vi "MetaData Channel.vi"(8 "error in (no error)":errorcluster, 11 "Node Ptr":T5 format="%.0x") -> (0 "error out":errorcluster)   [LabVIEW 2019, in "Instrument Addon System Explorer.lvlib"]
uses:
  Instrument Addon System Explorer.lvlib
  <vilib>/NI VeriStand/Custom Device API/Custom Device API.lvlib
  Addon Shared/Instrument Addon Shared.lvlib
  Addon Shared/Types/FG Control.ctl
  <vilib>/NI VeriStand/Custom Device API/Custom Device Channel Type.ctl
  <vilib>/NI VeriStand/Custom Device API/Custom Device Channel.ctl
  Addon Shared/Constants.vi
  <vilib>/NI VeriStand/Custom Device API/Custom Device Item Ref.ctl
  Addon Shared/Types/Protocol Data Type.ctl
  Addon Shared/Types/Metadata Channel Type.ctl
  Addon Shared/Types/Type Cast Type.ctl
  Addon Shared/Types/Endian.ctl
panel:
  in  "Delimiter":string=","
  in  "Reset":bool
  in  "Create":bool
  in  "Elements":u32
  in  "Units":string
  in  "Default Value":dbl
  out "Channel Type (Tab)":enum32{"List", "Format", "Type Cast"}(tab)
  in  "Remove":bool
  in  "Add":bool
  in  "Enumerated List":i32(listbox)
  in  "Test Value":dbl
  in  "Format String":string="%.3g"
  out "Validiated String":string
  in  "Endian":T1=enum."Little"
  in  "Type":T2
  in  "Channel Type":T3
  out "Data Type":T4
  in  "Header 2":cluster{"Section Name":string}={"Section Name"="MetaData Settings"}
  in  "SHDocVw.IWebBrowser":refnum<k7>(container)
  in  "Header":cluster{"Section Name":string}={"Section Name"="Custom Device Item Settings"}
  in  "Description":string
  in  "Name":string
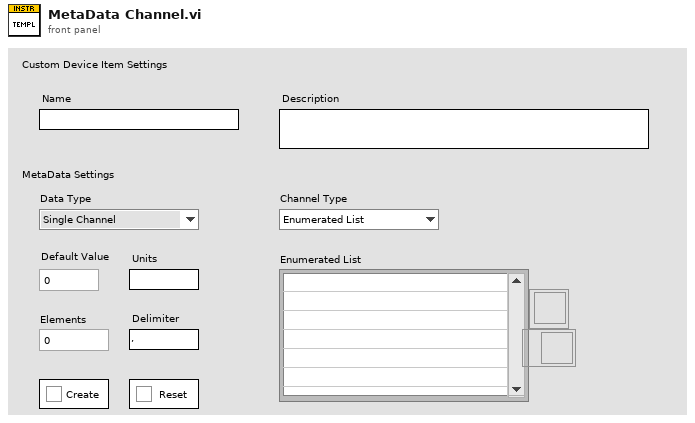
[diagram p1: front panel]
types:
  T1 = typedef "Instrument Addon Shared.lvlib/Endian.ctl" = enum16{"Native", "Little", "Big"}
  T2 = typedef "Instrument Addon Shared.lvlib/Type Cast Type.ctl" = enum16{"DBL", "SGL", "U64", "U32", "U16", "U8", "I64", "I32", "I16", "I8"}
  T3 = typedef "Instrument Addon Shared.lvlib/Metadata Channel Type.ctl" = enum16{"Enumerated List", "Format", "Type Cast"}
  T4 = typedef "Instrument Addon Shared.lvlib/Protocol Data Type.ctl" = enum16{"Single Channel", "Array"}
  T5 = typedef "Custom Device API.lvlib/Custom Device Item Ref.ctl" = u64
  T6 = typedef "Instrument Addon Shared.lvlib/FG Control.ctl" = enum16{"Get", "Set"}
  T7 = typedef "Custom Device API.lvlib/Custom Device Item Info.ctl" = cluster{"Name":string, "Is Channel":bool, "GUID":string, "Is Waveform":bool}
  T8 = typedef "Instrument Addon Shared.lvlib/MetaData Parameters.ctl" = cluster{"Data Type":T4, "Channel Type":T3, "List":string[], "Format String":string, "Type":T2, "Delimiter":string, "Endian":T1}
  T9 = typedef "Custom Device API.lvlib/Custom Device Channel.ctl" = cluster{"Type":T10, "Units":string, "Default Value":dbl, "Faultable":bool, "Scalable":bool}
  T10 = typedef "Custom Device API.lvlib/Custom Device Channel Type.ctl" = enum16{"Input", "Output"}
  T11 = typedef "Custom Device API.lvlib/Custom Device Commands.ctl" = enum16{"Default", "Item renamed", "Shutdown", "Dynamic button pressed"}
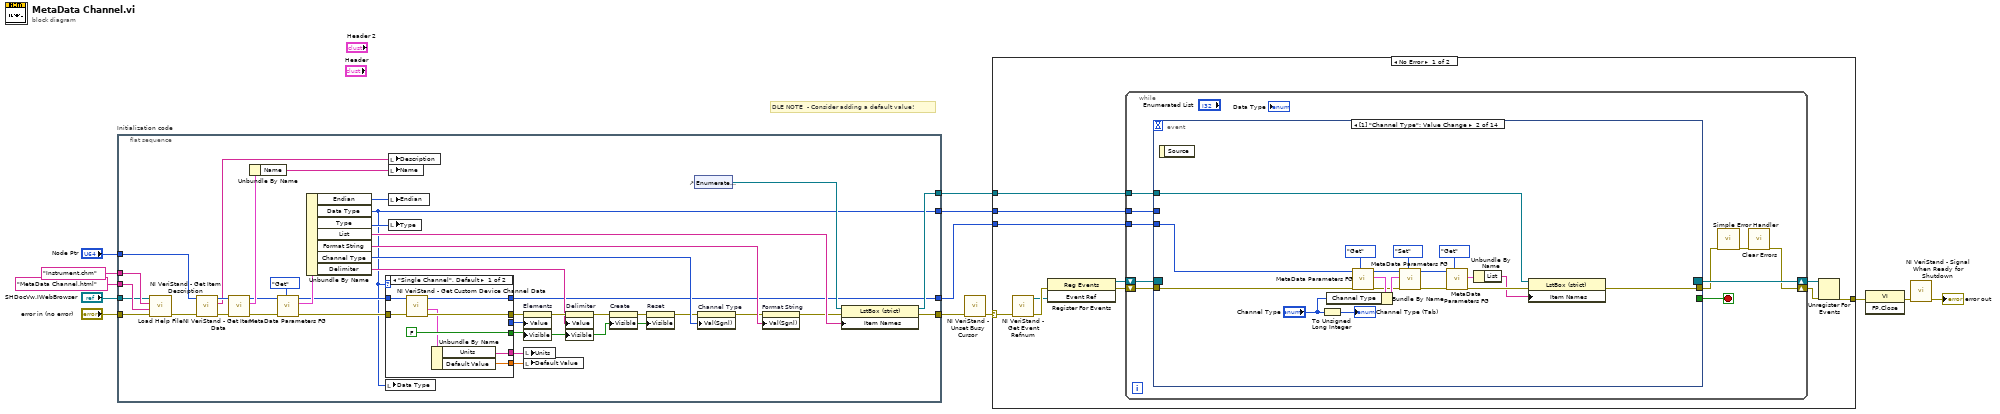
[diagram p0: block diagram]
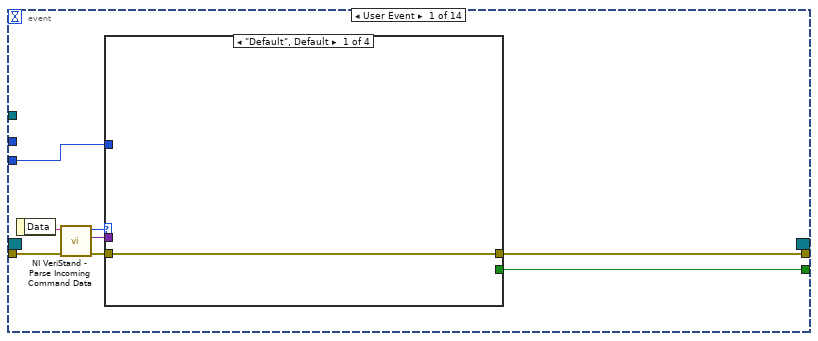
[diagram p2: hidden frame]
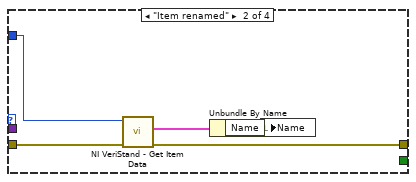
[diagram p3: hidden frame]
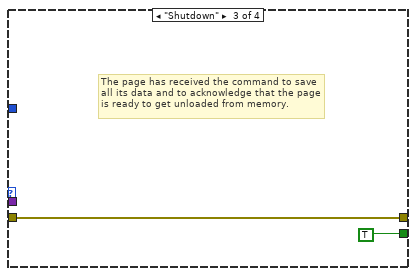
[diagram p4: hidden frame]
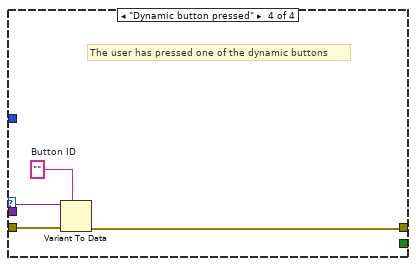
[diagram p5: hidden frame]
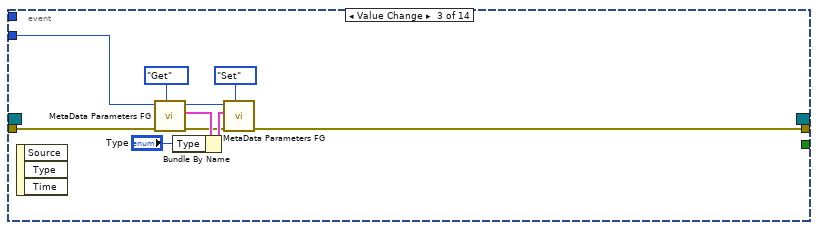
[diagram p6: hidden frame]
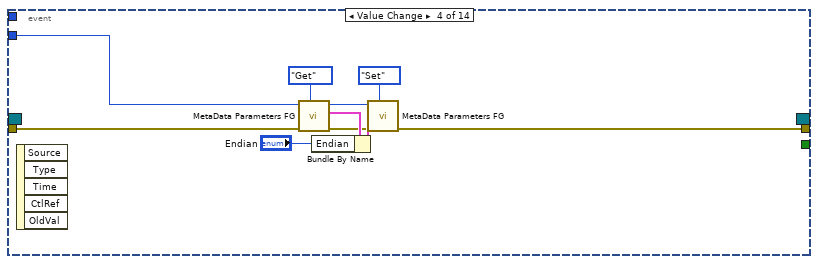
[diagram p7: hidden frame]
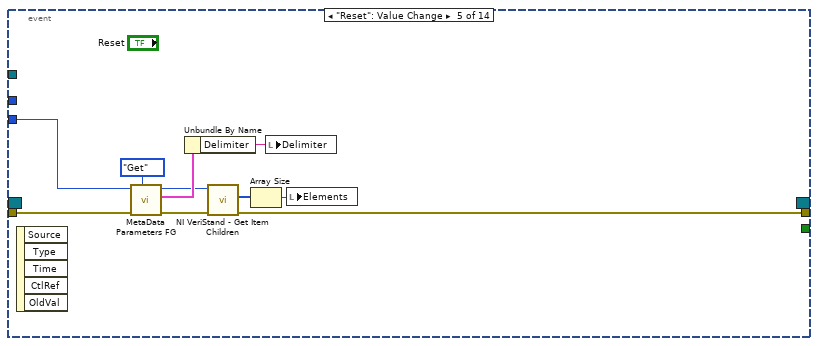
[diagram p8: hidden frame]
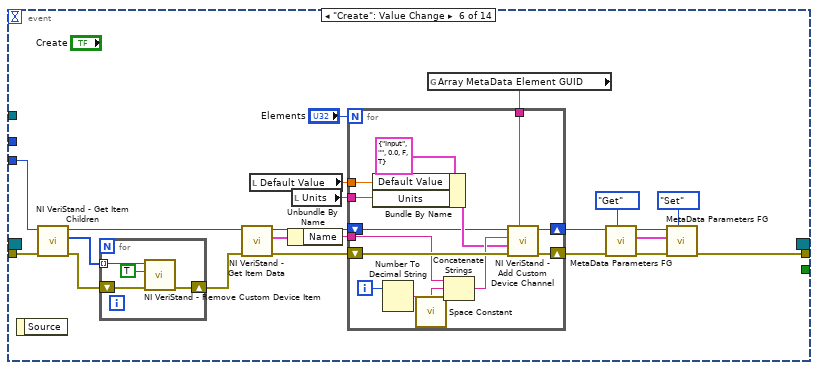
[diagram p9: hidden frame]
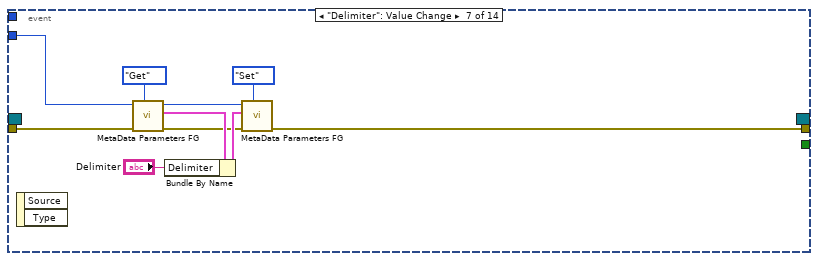
[diagram p10: hidden frame]
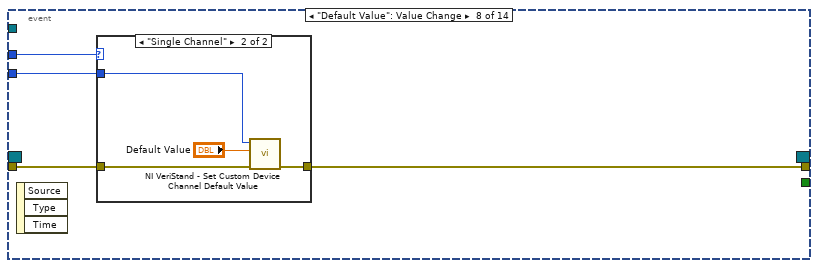
[diagram p11: hidden frame]
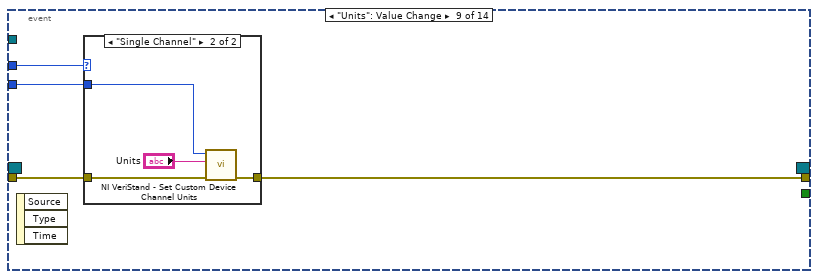
[diagram p13: hidden frame]
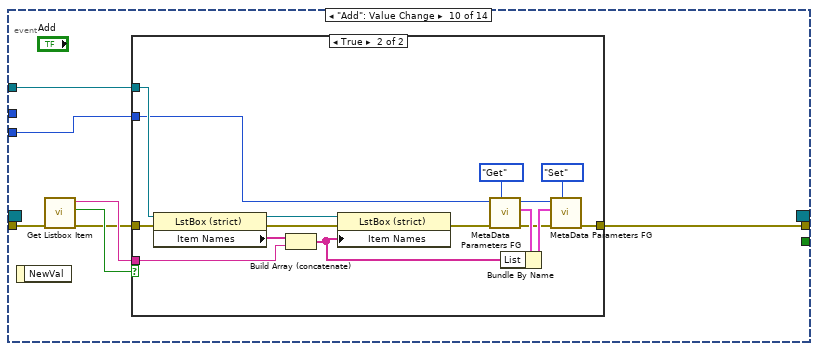
[diagram p15: hidden frame]
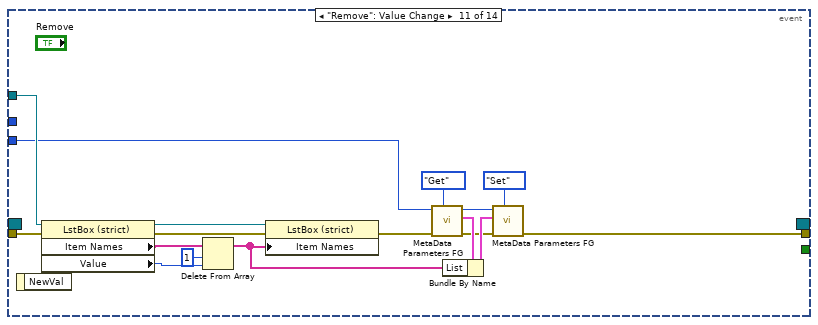
[diagram p17: hidden frame]
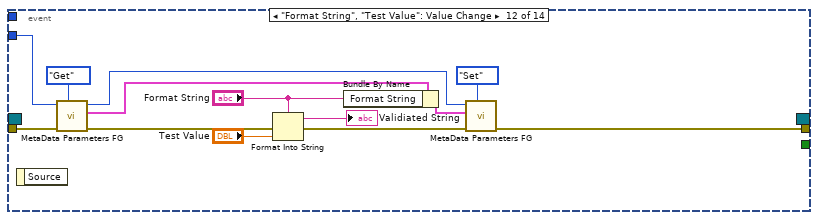
[diagram p18: hidden frame]
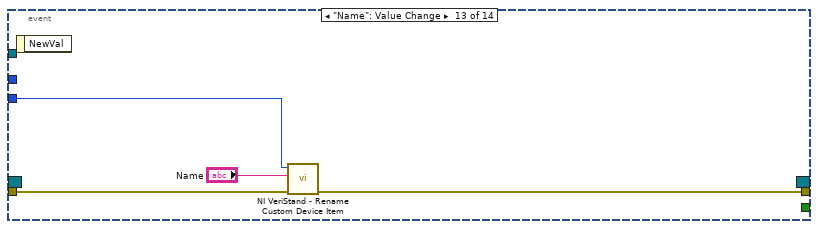
[diagram p19: hidden frame]
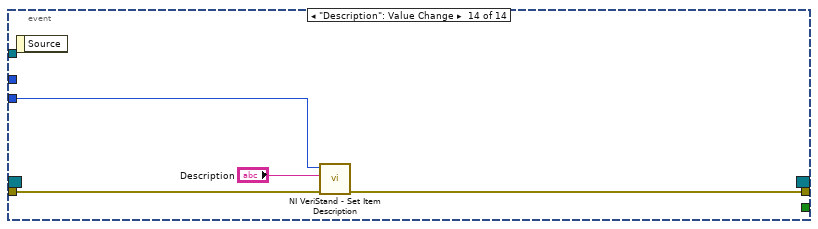
[diagram p20: hidden frame]
diagram:
  # "DLE NOTE  - Consider adding a default value!"
  n1 = flat-sequence "Initialization code" {
    tunnel: "error in (no error)" -> [w47]
    tunnel: "Node Ptr" -> [w32]
    tunnel: [w36] -> w9
    tunnel: [w20] -> w2
    tunnel: "Instrument.chm" ("Main CHM File") -> [w46]
    tunnel: "MetaData Channel.html" ("HTML File") -> [w45]
    tunnel: "SHDocVw.IWebBrowser" -> [w44]
    tunnel: [w34] -> w3
    tunnel: [w17] -> w1
    frame #0 {
      n2 = call "Load Help File.vi"("error in (no error)"=w47, "HTML File"=w45, "Main CHM File"=w46, "SHDocVw.IWebBrowser2"=w44) -> ("error out"=w33:errorcluster)  [unwired: 7 in]
      n3 = call <vilib>:"NI VeriStand - Get Item Description.vi"("error in (no error)"=w33, "Item Ref in"=w32) -> ("error out"=w50:errorcluster, "Description"=w51:string, "Item Ref out"=w52:T5)  [unwired: 7 out]
      n4 = call <vilib>:"NI VeriStand - Get Item Data.vi"("error in (no error)"=w50, "Item Ref in"=w52) -> ("error out"=w25:errorcluster, "Item Info"=w49:T7, "Item Ref out"=w24:T5)  [unwired: 7 out]
      n5 = Unbundle By Name(w49) -> ("Name"=w48:string)
      n6 = call "MetaData Parameters FG.vi"("Action"=FG_Control."Get", "error in (no error)"=w25, "Item Ref in"=w24) -> ("error out"=w23:errorcluster, "MetaData Parameters"=w42:T8, "Item Ref out"=w22:T5)  [unwired: 6 in]
      n7 = Unbundle By Name(w42) -> ("Endian"=w15:T1, "Data Type"=w17:T4, "Type"=w31:T2, "List"=w40:string[], "Format String"=w39:string, "Channel Type"=w41:T3, "Delimiter"=w26:string)
      n8 = case shown="\"Single Channel\", Default" w17 {
        tunnel: [FALSE TRUE] -> w14
        tunnel: w23 -> [w59 w64]
        tunnel: w22 -> [w58 w68]
        tunnel: [w57 w63] -> w21
        tunnel: [w56 w65] -> w20
        tunnel: [w54 ""] -> w19
        tunnel: [w53 0.0 ("Default Value")] -> w18
        tunnel: [_ w61] -> w16
        frame "Single Channel", Default {
          n9 = call <vilib>:"NI VeriStand - Get Custom Device Channel Data.vi"("error in (no error)"=w59, "Channel Ref in"=w58) -> ("error out"=w57:errorcluster, "Channel"=w55:T9, "Channel Ref out"=w56:T5)  [unwired: 4 in, 3 out]
          n10 = Unbundle By Name(w55) -> ("Units"=w54:string, "Default Value"=w53:dbl)
        }
        frame "Array" {
          n11 = call <vilib>:"NI VeriStand - Get Item Children.vi"("error in (no error)"=w64, "Item Ref in"=w68) -> ("error out"=w63:errorcluster, "Child Refs"=w62:T5[], "Item Ref out"=w65:T5)  [unwired: 6 in, 1 out]
          n12 = Array Size(array=w62) -> (size(s)=w61:i32)
        }
      }
      n13 = local write "Data Type"(w17) -> ()
      n14 = local write "Description"(w51) -> ()
      n15 = local write "Name"(w48) -> ()
      n16 = local write "Endian"(w15) -> ()
      n17 = local write "Type"(w31) -> ()
      n18 = property on="Elements" class="DigNum (strict)"(error in=w21, "Value"=w16, "Visible"=w14) -> (error out=w28:errorcluster)  [unwired: 1 in, 1 out]
      n19 = local write "Units"(w19) -> ()
      n20 = local write "Default Value"(w18) -> ()
      n21 = property on="Delimiter" class="Str"(error in=w28, "Value"=w26, "Visible"=w14) -> (error out=w29:errorcluster)  [unwired: 1 in, 1 out]
      n22 = property on="Create" class="Bool"(error in=w29, "Visible"=w14) -> (error out=w30:errorcluster)  [unwired: 1 in, 1 out]
      n23 = property on="Reset" class="Bool"(error in=w30, "Visible"=w14) -> (error out=w27:errorcluster)  [unwired: 1 in, 1 out]
      n24 = control-ref of="Enumerated List"() -> (w35:refnum<vi>)
      n25 = property on="Channel Type" class="Enum (strict)"(error in=w27, "Val(Sgnl)"=w41) -> (error out=w38:errorcluster)  [unwired: 1 in, 1 out]
      n26 = property on="Format String" class="Str"(error in=w38, "Val(Sgnl)"=w39) -> (error out=w37:errorcluster)  [unwired: 1 in, 1 out]
      n27 = property class="LstBox (strict)"(reference=w35, error in=w37, "Item Names"=w40) -> (reference out=w34:refnum<vi>, error out=w36:errorcluster)
    }
  }
  n28 = call <vilib>:"NI VeriStand - Unset Busy Cursor.vi"("error in (no error)"=w9) -> ("error out"=w8:errorcluster)  [unwired: 10 out]
  n29 = case shown="No Error" w8 {
    selector: w8 -> [w72 w291]
    tunnel: [w77 w289] -> w13
    tunnel: w2 -> [w73 _]
    tunnel: w3 -> [w71 _]
    tunnel: w1 -> [w70 _]
    frame No Error {
      n30 = call <vilib>:"NI VeriStand - Get Event Refnum.vi"("error in (no error)"=w72) -> ("error out"=w80:errorcluster, "Event Ref"=w76:refnum<user-event>)  [unwired: 9 out]
      n31 = register-events(error in=w80, w76) -> (reference out=w74:refnum<event-registration>, error out=w75:errorcluster)  [unwired: 1 in]
      n32 = while {
        tunnel: w73 -> [w86]
        shift-right: [w83] -> w78
        shift-left: w75 -> [w89]
        shift-right: [w90] -> w79
        shift-left: w74 -> [w88]
        tunnel: w71 -> [w82]
        tunnel: w70 -> [w81]
        stop <- w87 stop-if-true
        n33 = event shown="[1] \"Channel Type\": Value Change" {
          selector: w88 -> [_ _ _ _ _ _ _ _ _ _ _ _ _ _]
          dyn-events: [_ _ _ _ _ _ _ _ _ _ _ _ _ _] -> w90
          timeout: _ -> [_ _ _ _ _ _ _ _ _ _ _ _ _ _]
          tunnel: w89 -> [w98 w122 w133 w143 w156 w170 w201 w212 w221 w228 w264 w276 w284 w287]
          tunnel: [w94 _ _ _ _ _ _ _ _ _ _ _ _ _] -> w87
          tunnel: [w93 w111 w129 w140 w150 w160 w199 w211 w220 w232 w253 w277 w283 w286] -> w85
          tunnel: w86 -> [w92 w121 w132 w142 w155 w179 w200 w210 w219 w231 w251 w274 w282 w288]
          tunnel: w82 -> [_ w113 _ _ _ _ _ _ _ w233 w267 _ _ _]
          tunnel: w81 -> [_ _ _ _ _ _ _ w209 w218 _ _ _ _ _]
          event User Event {
            n34 = event-data() -> ("Data"=w97:string)  [unwired: 1 out]
            n35 = call <vilib>:"NI VeriStand - Parse Incoming Command Data.vi"("error in (no error)"=w98, "Incoming data"=w97) -> ("error out"=w96:errorcluster, "Outgoing data"=w91:variant, "Action"=w95:T11)  [unwired: 7 out]
            n36 = case shown="\"Default\", Default" w95 {
              tunnel: w96 -> [w99 w104 w105 w110]
              tunnel: [_ _ TRUE _] -> w94
              tunnel: [w99 w101 w105 w107] -> w93
              tunnel: w92 -> [_ w103 _ _]
              tunnel: w91 -> [_ _ _ w109]
              frame "Default", Default {
              }
              frame "Item renamed" {
                n37 = call <vilib>:"NI VeriStand - Get Item Data.vi"("error in (no error)"=w104, "Item Ref in"=w103) -> ("error out"=w101:errorcluster, "Item Info"=w102:T7)  [unwired: 8 out]
                n38 = Unbundle By Name(w102) -> ("Name"=w100:string)
                n39 = local write "Name"(w100) -> ()
              }
              frame "Shutdown" {
                # "The page has received the command to save all its data and to acknowledge that the page is ready to get unloaded from memory."
              }
              frame "Dynamic button pressed" {
                w108 = ""  # Button ID
                # "The user has pressed one of the dynamic buttons"
                n40 = Variant To Data(error in=w110, type=w108, Variant=w109) -> (error out=w107:errorcluster)  [unwired: 1 out]
              }
            }
          }
          event Value Change {
            n41 = event-data() -> ()  [unwired: 2 out]
            n42 = To Unsigned Long Integer(number="Channel Type") -> (unsigned 32bit integer=→"Channel Type (Tab)":u32)
            n43 = call "MetaData Parameters FG.vi"("Action"=FG_Control."Get", "error in (no error)"=w122, "Item Ref in"=w121) -> ("error out"=w120:errorcluster, "MetaData Parameters"=w126:T8, "Item Ref out"=w124:T5)  [unwired: 6 in]
            n44 = Bundle By Name(cluster=w126, "Channel Type"="Channel Type") -> (w125:T8)
            n45 = call "MetaData Parameters FG.vi"("Action"=FG_Control."Set", "error in (no error)"=w120, "MetaData Parameters"=w125, "Item Ref in"=w124) -> ("error out"=w115:errorcluster, "Item Ref out"=w114:T5)  [unwired: 5 in, 1 out]
            n46 = call "MetaData Parameters FG.vi"("Action"=FG_Control."Get", "error in (no error)"=w115, "Item Ref in"=w114) -> ("error out"=w117:errorcluster, "MetaData Parameters"=w118:T8)  [unwired: 6 in, 1 out]
            n47 = Unbundle By Name(w118) -> ("List"=w116:string[])
            n48 = property class="LstBox (strict)"(reference=w113, error in=w117, "Item Names"=w116) -> (error out=w111:errorcluster)  [unwired: 1 out]
          }
          event Value Change {
            n49 = event-data() -> ()  [unwired: 4 out]
            n50 = call "MetaData Parameters FG.vi"("Action"=FG_Control."Get", "error in (no error)"=w133, "Item Ref in"=w132) -> ("error out"=w131:errorcluster, "MetaData Parameters"=w137:T8, "Item Ref out"=w135:T5)  [unwired: 6 in]
            n51 = Bundle By Name(cluster=w137, "Type"="Type") -> (w136:T8)
            n52 = call "MetaData Parameters FG.vi"("Action"=FG_Control."Set", "error in (no error)"=w131, "MetaData Parameters"=w136, "Item Ref in"=w135) -> ("error out"=w129:errorcluster)  [unwired: 5 in, 2 out]
          }
          event Value Change {
            n53 = event-data() -> ()  [unwired: 6 out]
            n54 = call "MetaData Parameters FG.vi"("Action"=FG_Control."Get", "error in (no error)"=w143, "Item Ref in"=w142) -> ("error out"=w141:errorcluster, "MetaData Parameters"=w147:T8, "Item Ref out"=w145:T5)  [unwired: 6 in]
            n55 = Bundle By Name(cluster=w147, "Endian"="Endian") -> (w146:T8)
            n56 = call "MetaData Parameters FG.vi"("Action"=FG_Control."Set", "error in (no error)"=w141, "MetaData Parameters"=w146, "Item Ref in"=w145) -> ("error out"=w140:errorcluster)  [unwired: 5 in, 2 out]
          }
          event "Reset": Value Change {
            n57 = event-data() -> ()  [unwired: 6 out]
            n58 = call "MetaData Parameters FG.vi"("Action"=FG_Control."Get", "error in (no error)"=w156, "Item Ref in"=w155) -> ("error out"=w151:errorcluster, "MetaData Parameters"=w158:T8, "Item Ref out"=w152:T5)  [unwired: 6 in]
            n59 = Unbundle By Name(w158) -> ("Delimiter"=w154:string)
            n60 = call <vilib>:"NI VeriStand - Get Item Children.vi"("error in (no error)"=w151, "Item Ref in"=w152) -> ("error out"=w150:errorcluster, "Child Refs"=w153:T5[])  [unwired: 6 in, 2 out]
            n61 = Array Size(array=w153) -> (size(s)=w149:i32)
            n62 = local write "Delimiter"(w154) -> ()
            n63 = local write "Elements"(w149) -> ()
          }
          event "Create": Value Change {
            n64 = event-data() -> ()  [unwired: 2 out]
            n65 = call <vilib>:"NI VeriStand - Get Item Children.vi"("error in (no error)"=w170, "Item Ref in"=w179) -> ("error out"=w167:errorcluster, "Child Refs"=w168:T5[], "Item Ref out"=w171:T5)  [unwired: 6 in, 1 out]
            n66 = for {
              shift-right: [w183] -> w169
              shift-left: w167 -> [w181]
              tunnel: w168 -> [w182] mode=indexing
              n67 = call <vilib>:"NI VeriStand - Remove Custom Device Item.vi"("error in (no error)"=w181, "Force Delete (F)"=TRUE, "Item Ref in"=w182) -> ("error out"=w183:errorcluster)  [unwired: 7 in, 1 out]
            }
            n68 = call <vilib>:"NI VeriStand - Get Item Data.vi"("error in (no error)"=w169, "Item Ref in"=w171) -> ("error out"=w178:errorcluster, "Item Info"=w180:T7, "Item Ref out"=w172:T5)  [unwired: 7 out]
            n69 = local read "Default Value"() -> (w175:dbl)
            n70 = Unbundle By Name(w180) -> ("Name"=w177:string)
            n71 = local read "Units"() -> (w176:string)
            n72 = global read "Constants.vi" "Array MetaData Element GUID"() -> (w173:string)
            n73 = for {
              N: "Elements" -> [_]
              shift-right: [w197] -> w161
              shift-left: w178 -> [w198]
              tunnel: w177 -> [w195]
              tunnel: w176 -> [w189]
              tunnel: w175 -> [w188]
              tunnel: w173 -> [w187]
              shift-right: [w185] -> w159
              shift-left: w172 -> [w186]
              i -> [w196]
              n74 = Bundle By Name(cluster=T9 {"Type"=enum."Input", "Units"="", "Default Value"=0.0, "Faultable"=FALSE, "Scalable"=TRUE} ("Channel"), "Default Value"=w188, "Units"=w189) -> (w190:T9)
              n75 = Number To Decimal String(number=w196) -> (decimal integer string=w194:string)  [unwired: 1 in]
              n76 = call <vilib>:"Space Constant.vi"() -> ("String"=w193:string)
              n77 = Concatenate Strings(w195, w193, w194) -> (w192:string)
              n78 = call <vilib>:"NI VeriStand - Add Custom Device Channel.vi"("GUID (Default Channel)"=w187, "error in (no error)"=w198, "Channel"=w190, "Channel Name"=w192, "Parent Ref in"=w186) -> ("error out"=w197:errorcluster, "Parent Ref out"=w185:T5)  [unwired: 3 in, 2 out]
            }
            n79 = call "MetaData Parameters FG.vi"("Action"=FG_Control."Get", "error in (no error)"=w161, "Item Ref in"=w159) -> ("error out"=w163:errorcluster, "MetaData Parameters"=w162:T8, "Item Ref out"=w165:T5)  [unwired: 6 in]
            n80 = call "MetaData Parameters FG.vi"("Action"=FG_Control."Set", "error in (no error)"=w163, "MetaData Parameters"=w162, "Item Ref in"=w165) -> ("error out"=w160:errorcluster)  [unwired: 5 in, 2 out]
          }
          event "Delimiter": Value Change {
            n81 = event-data() -> ()  [unwired: 3 out]
            n82 = call "MetaData Parameters FG.vi"("Action"=FG_Control."Get", "error in (no error)"=w201, "Item Ref in"=w200) -> ("error out"=w204:errorcluster, "MetaData Parameters"=w208:T8, "Item Ref out"=w206:T5)  [unwired: 6 in]
            n83 = Bundle By Name(cluster=w208, "Delimiter"="Delimiter") -> (w207:T8)
            n84 = call "MetaData Parameters FG.vi"("Action"=FG_Control."Set", "error in (no error)"=w204, "MetaData Parameters"=w207, "Item Ref in"=w206) -> ("error out"=w199:errorcluster)  [unwired: 5 in, 2 out]
          }
          event "Default Value": Value Change {
            n85 = event-data() -> ()  [unwired: 4 out]
            n86 = case shown="\"Single Channel\"" w209 {
              tunnel: w212 -> [w213 w217]
              tunnel: [w213 w216] -> w211
              tunnel: w210 -> [_ w215]
              frame "Array" {
              }
              frame "Single Channel" {
                n87 = call <vilib>:"NI VeriStand - Set Custom Device Channel Default Value.vi"("error in (no error)"=w217, "Default Value"="Default Value", "Channel Ref in"=w215) -> ("error out"=w216:errorcluster)  [unwired: 7 in, 1 out]
              }
            }
          }
          event "Units": Value Change {
            n88 = event-data() -> ()  [unwired: 4 out]
            n89 = case shown="\"Single Channel\"" w218 {
              tunnel: w221 -> [w222 w226]
              tunnel: [w222 w225] -> w220
              tunnel: w219 -> [_ w224]
              frame "Array" {
              }
              frame "Single Channel" {
                n90 = call <vilib>:"NI VeriStand - Set Custom Device Channel Units.vi"("error in (no error)"=w226, "Units"="Units", "Channel Ref in"=w224) -> ("error out"=w225:errorcluster)  [unwired: 7 in, 1 out]
              }
            }
          }
          event "Add": Value Change {
            n91 = event-data() -> ()  [unwired: 2 out]
            n92 = call "Get Listbox Item.vi"("error in (no error)"=w228) -> ("error out"=w227:errorcluster, "OK?"=w229:bool, "Item out"=w230:string)  [unwired: 8 in]
            n93 = case shown="True" w229 {
              tunnel: w233 -> [_ w250]
              tunnel: w227 -> [w234 w249]
              tunnel: w230 -> [_ w245]
              tunnel: [w234 w236] -> w232
              tunnel: w231 -> [_ w238]
              frame False {
              }
              frame True {
                n94 = property class="LstBox (strict)"(reference=w250, error in=w249) -> (reference out=w248:refnum<vi>, error out=w247:errorcluster, "Item Names"=w246:string[])
                n95 = Build Array (concatenate)(w246, w245) -> (w235:string[])
                n96 = property class="LstBox (strict)"(reference=w248, error in=w247, "Item Names"=w235) -> (error out=w237:errorcluster)  [unwired: 1 out]
                n97 = call "MetaData Parameters FG.vi"("Action"=FG_Control."Get", "error in (no error)"=w237, "Item Ref in"=w238) -> ("error out"=w239:errorcluster, "MetaData Parameters"=w243:T8, "Item Ref out"=w241:T5)  [unwired: 6 in]
                n98 = Bundle By Name(cluster=w243, "List"=w235) -> (w242:T8)
                n99 = call "MetaData Parameters FG.vi"("Action"=FG_Control."Set", "error in (no error)"=w239, "MetaData Parameters"=w242, "Item Ref in"=w241) -> ("error out"=w236:errorcluster)  [unwired: 5 in, 2 out]
              }
            }
          }
          event "Remove": Value Change {
            n100 = event-data() -> ()  [unwired: 2 out]
            n101 = property class="LstBox (strict)"(reference=w267, error in=w264) -> (reference out=w266:refnum<vi>, error out=w265:errorcluster, "Item Names"=w263:string[], "Value"=w262:i32)
            n102 = Delete From Array(array=w263, length=1, index=w262) -> (array with subset deleted=w252:string[])  [unwired: 1 out]
            n103 = property class="LstBox (strict)"(reference=w266, error in=w265, "Item Names"=w252) -> (error out=w254:errorcluster)  [unwired: 1 out]
            n104 = call "MetaData Parameters FG.vi"("Action"=FG_Control."Get", "error in (no error)"=w254, "Item Ref in"=w251) -> ("error out"=w255:errorcluster, "MetaData Parameters"=w259:T8, "Item Ref out"=w257:T5)  [unwired: 6 in]
            n105 = Bundle By Name(cluster=w259, "List"=w252) -> (w258:T8)
            n106 = call "MetaData Parameters FG.vi"("Action"=FG_Control."Set", "error in (no error)"=w255, "MetaData Parameters"=w258, "Item Ref in"=w257) -> ("error out"=w253:errorcluster)  [unwired: 5 in, 2 out]
          }
          event "Format String", "Test Value": Value Change {
            n107 = event-data() -> ()  [unwired: 2 out]
            n108 = call "MetaData Parameters FG.vi"("Action"=FG_Control."Get", "error in (no error)"=w276, "Item Ref in"=w274) -> ("error out"=w275:errorcluster, "MetaData Parameters"=w272:T8, "Item Ref out"=w269:T5)  [unwired: 6 in]
            n109 = Format Into String(format string="Format String", error in=w275, "Test Value") -> (resulting string=→"Validiated String":string, error out=w278:errorcluster)  [unwired: 1 in]
            n110 = Bundle By Name(cluster=w272, "Format String"="Format String") -> (w270:T8)
            n111 = call "MetaData Parameters FG.vi"("Action"=FG_Control."Set", "error in (no error)"=w278, "MetaData Parameters"=w270, "Item Ref in"=w269) -> ("error out"=w277:errorcluster)  [unwired: 5 in, 2 out]
          }
          event "Name": Value Change {
            n112 = event-data() -> ()  [unwired: 2 out]
            n113 = call <vilib>:"NI VeriStand - Rename Custom Device Item.vi"("error in (no error)"=w284, "New Name"="Name", "Item Ref in"=w282) -> ("error out"=w283:errorcluster)  [unwired: 1 in, 7 out]
          }
          event "Description": Value Change {
            n114 = event-data() -> ()  [unwired: 2 out]
            n115 = call <vilib>:"NI VeriStand - Set Item Description.vi"("error in (no error)"=w287, "Description"="Description", "Item Ref in"=w288) -> ("error out"=w286:errorcluster)  [unwired: 8 out]
          }
        }
        n116 = call <vilib>:"Simple Error Handler.vi"("error in (no error)"=w85) -> ("error out"=w84:errorcluster)  [unwired: 1 in, 7 out]
        n117 = call <vilib>:"Clear Errors.vi"("error in (no error)"=w84) -> ("error out"=w83:errorcluster)  [unwired: 1 in, 5 out]
      }
      n118 = Unregister For Events(event registration refnum=w79, error in=w78) -> (error out=w77:errorcluster)
    }
    frame Error {
      n119 = call <vilib>:"Simple Error Handler.vi"("error in (no error)"=w291) -> ("error out"=w290:errorcluster)  [unwired: 1 in, 7 out]
      n120 = call <vilib>:"Clear Errors.vi"("error in (no error)"=w290) -> ("error out"=w289:errorcluster)  [unwired: 1 in, 5 out]
    }
  }
  n121 = invoke class="VI" method="FP.Close"(error in=w13) -> (error out=w12:errorcluster)  [unwired: 2 in, 2 out]
  n122 = call <vilib>:"NI VeriStand - Signal When Ready for Shutdown.vi"("error in (no error)"=w12) -> ("error out"=→"error out":errorcluster)  [unwired: 10 out]
